vi "Main.vi"(11 "Module Admin":refnum<class "Delacor_lib_QMH_Module Admin.lvclass">) -> ()   [LabVIEW 2020, in "Topas.lvlib"]
doc: "This template is based off of the Queued Message Handler design pattern and the Queued Message Handler project template that ships with LabVIEW.\n\nThe main difference is that the queue is private to this module and communication between modules is performed via Broadcast and Request events.\n\nRequest events are wrapped in public API methods and are handled in the Event Handling Loop (EHL) of this VI. Any module can register for Broadcast events sent by this module. The EHL generates messages based on user interface actions.\n\nThe Message Handling Loop (MHL) processes messages generated by the EHL, or by other messages. The messages are string values, so new messages can be added easily to the Message Cases case structure in the MHL. Each message cluster can also provide an optional value for Message Data, which is a variant that can be converted to whatever message-specific data is required.\n_____\nBased on Delacor QMH Project Template 5.0.0.82."
uses:
  Topas.lvlib
  <vilib>/Delacor/Delacor QMH/Libraries/Module Admin_class/Delacor_lib_QMH_Module Admin.lvclass
  Module Data--cluster.ctl
  Topas-LVClass/Abstract Topas/Abstract Topas.lvclass
  Stop Argument--cluster.ctl
  <vilib>/Delacor/Delacor QMH/Libraries/Message Queue_class/Delacor_lib_QMH_Message Queue.lvclass/Delacor_lib_QMH_Message Queue.ctl
  <vilib>/Delacor/Delacor QMH/Libraries/Module Admin_class/Delacor_lib_QMH_Module Admin.lvclass/Delacor_lib_QMH_Module Admin.ctl
  Set Wavelength Argument--cluster.ctl
  Set Wavelength (Reply Payload)--cluster.ctl
  Open Shutter Argument--cluster.ctl
  Get Wavelength Argument--cluster.ctl
  Get Wavelength (Reply Payload)--cluster.ctl
  Get Module Data Argument--cluster.ctl
  Get Module Data (Reply Payload)--cluster.ctl
  <vilib>/Utility/miscctls.llb/LVPointTypeDef.ctl
  <vilib>/Delacor/Delacor QMH/Libraries/Message Queue_class/Delacor_lib_QMH_Enqueue Message (Single).vi
  <vilib>/Delacor/Delacor QMH/Libraries/Module Admin_class/Delacor_lib_QMH_Get External Launch.vi
  <vilib>/Utility/error.llb/Error Cluster From Error Code.vi
  <vilib>/ErrorRing/Error Ring.xnode
  <vilib>/Delacor/Delacor QMH/Libraries/Message Queue_class/Delacor_lib_QMH_Message Queue.lvclass
panel:
  out "error out":errorcluster
  out "Status":string
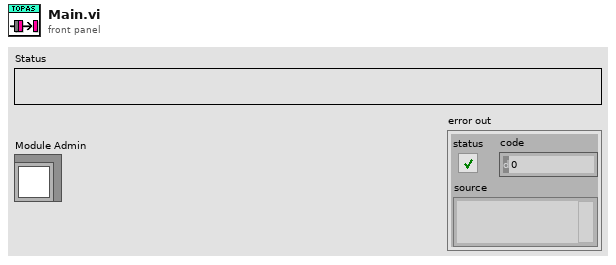
[diagram p1: front panel]
types:
  T1 = typedef "Topas.lvlib/Request Events--cluster.ctl" = cluster{"Stop Module":refnum<user-event>, "Show Panel":refnum<user-event>, "Hide Panel":refnum<user-event>, "Get Module Execution Status":refnum<user-event>, "Show Diagram":refnum<user-event>, "Set Wavelength":refnum<user-event>, "Open Shutter":refnum<user-event>, "Get Wavelength":refnum<user-event>, "Get Module Data":refnum<user-event>}
  T2 = typedef "Topas.lvlib/Module Data--cluster.ctl" = cluster{"Status":string, "Wavelength":dbl, "-Topas Class":refnum<class "Abstract Topas.lvclass">}
  T3 = enum32{"invalid lock state", "Not Locked", "Locked (No Password)", "Password-protected"}
  T4 = typedef "Topas.lvlib/Stop Argument--cluster.ctl" = cluster{"Origin":string, "Exit via Stop Module Req?":bool, "Wait for Module to stop?":bool}
  T5 = typedef "Topas.lvlib/Set Wavelength Argument--cluster.ctl" = cluster{"Wavelength":dbl, "Wait Notifier":refnum<notifier>, "wait for reply":bool}
  T6 = typedef "Topas.lvlib/Open Shutter Argument--cluster.ctl" = cluster{"Open Shutter":bool}
  T7 = typedef "Topas.lvlib/Get Wavelength Argument--cluster.ctl" = cluster{"Wait Notifier":refnum<notifier>, "wait for reply":bool}
  T8 = typedef "Topas.lvlib/Get Module Data Argument--cluster.ctl" = cluster{"Wait Notifier":refnum<notifier>, "wait for reply":bool}
  T9 = typedef "LVPointTypeDef.ctl" = cluster{"Horizontal":i16, "Vertical":i16}
  T10 = enum32{"Invalid", "Standard", "Closed", "Hidden", "Minimized", "Maximized"}
  T11 = typedef "Topas.lvlib/Set Wavelength (Reply Payload)--cluster.ctl" = cluster{"Wavelength":dbl, "Set Wavelength_error":errorcluster}
  T12 = typedef "Topas.lvlib/Get Wavelength (Reply Payload)--cluster.ctl" = cluster{"Wavelength":dbl, "Get Wavelength_error":errorcluster}
  T13 = typedef "Topas.lvlib/Get Module Data (Reply Payload)--cluster.ctl" = cluster{"Topas":T2, "Get Module Data_error":errorcluster}
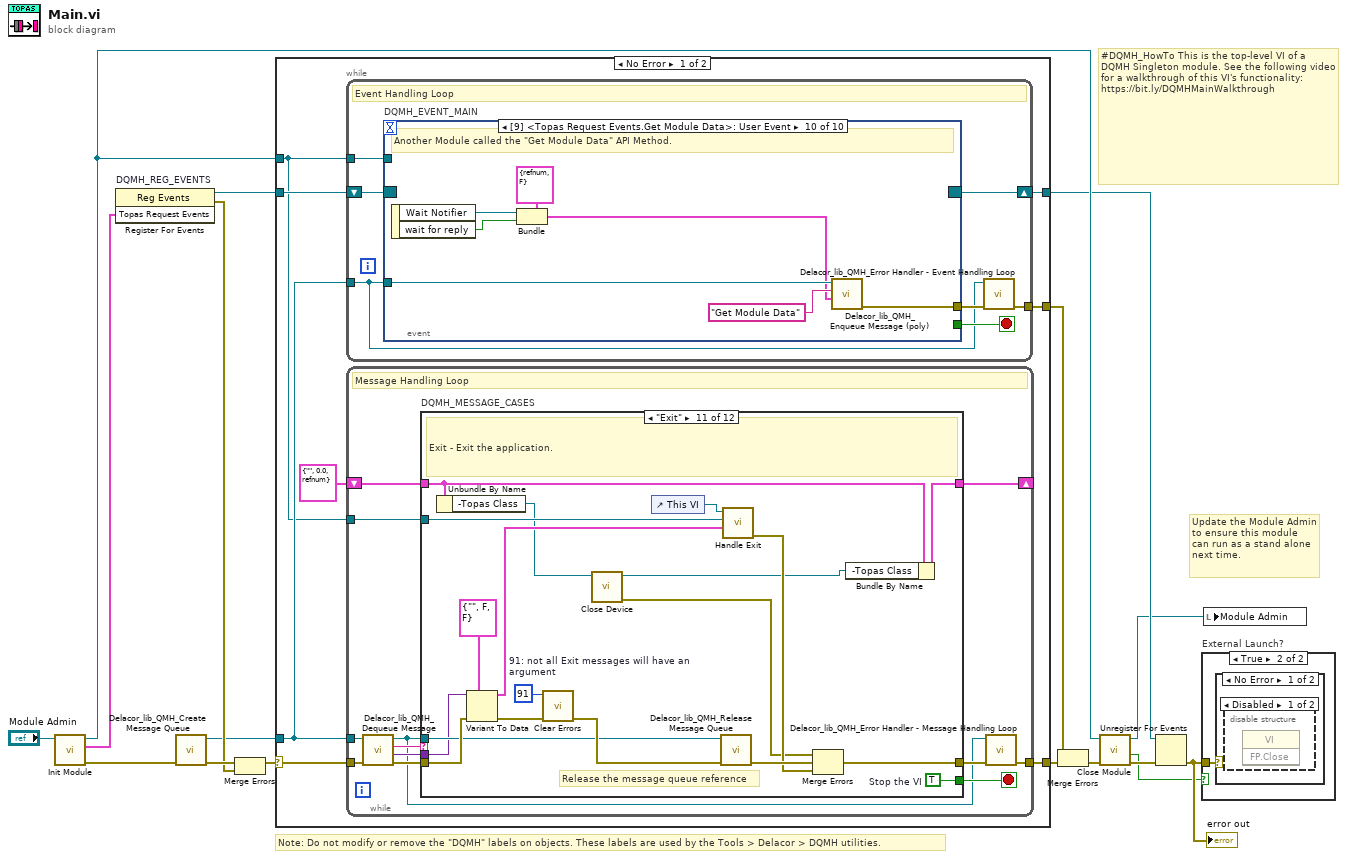
[diagram p0: block diagram]
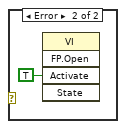
[diagram p4: hidden frame]
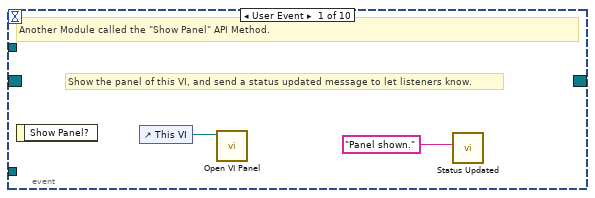
[diagram p5: hidden frame]
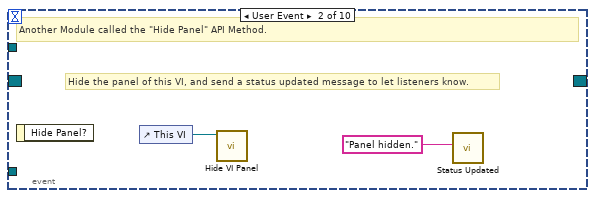
[diagram p6: hidden frame]
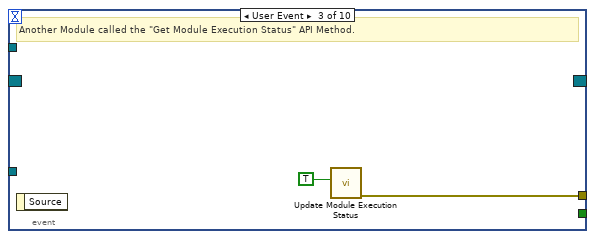
[diagram p7: hidden frame]
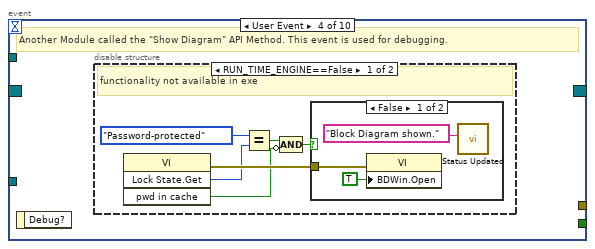
[diagram p8: hidden frame]
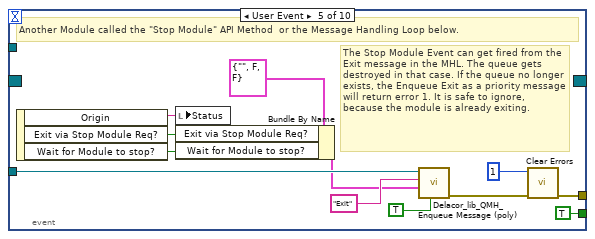
[diagram p11: hidden frame]
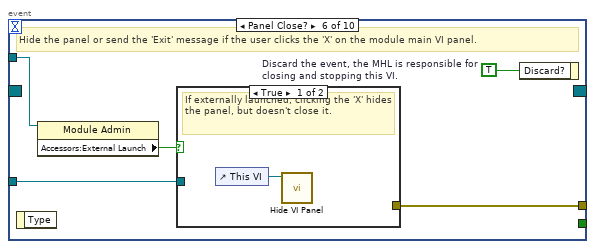
[diagram p12: hidden frame]
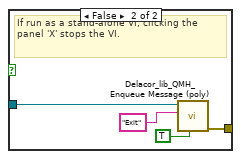
[diagram p13: hidden frame]
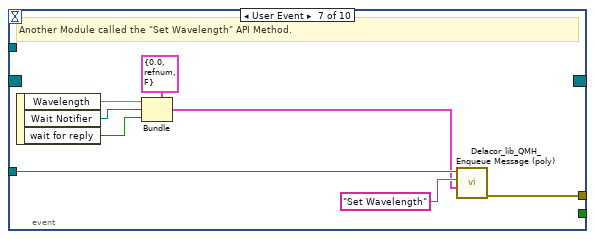
[diagram p14: hidden frame]
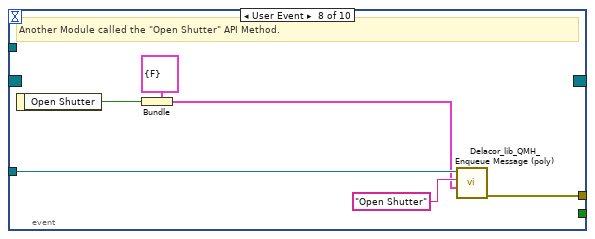
[diagram p15: hidden frame]
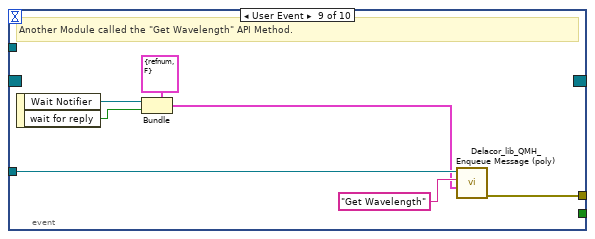
[diagram p16: hidden frame]
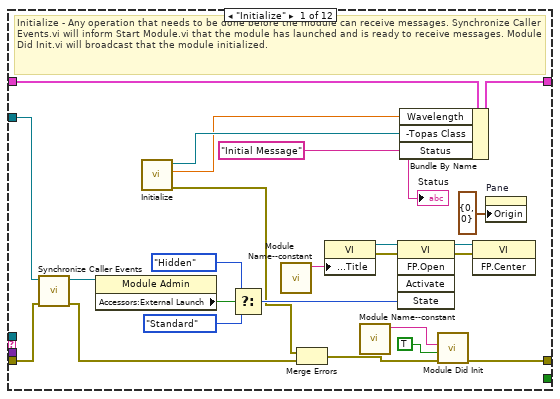
[diagram p17: hidden frame]
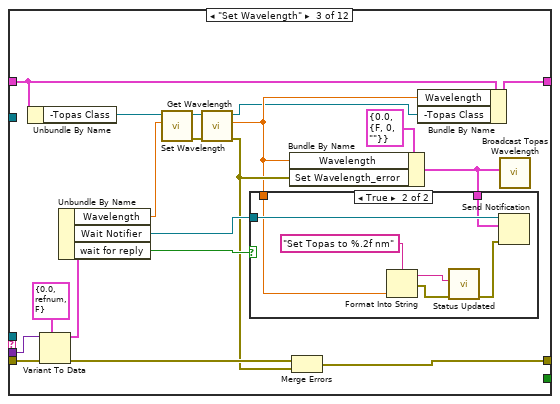
[diagram p19: hidden frame]
diagram:
  # "#DQMH_HowTo This is the top-level VI of a DQMH Singleton module. See the following video for a walkthrough of this VI's functionality: https://bit.ly/DQMHMainWalkthrough"
  # "Note: Do not modify or remove the \"DQMH\" labels on objects. These labels are used by the Tools > Delacor > DQMH utilities."
  # "Update the Module Admin to ensure this module can run as a stand alone next time."
  n1 = call "Init Module.vi"("Singleton Module Admin in"="Module Admin") -> ("error out"=w16:errorcluster, "Topas Request Events"=w5:T1, "Singleton Module Admin out"=w8:refnum<class "Delacor_lib_QMH_Module Admin.lvclass">)  [unwired: 8 in]
  n2 = register-events "DQMH_REG_EVENTS"(w5) -> (reference out=w6:refnum<event-registration>, error out=w9:errorcluster)  [unwired: 2 in]
  n3 = call <vilib>:"Delacor_lib_QMH_Create Message Queue.vi"("error in (no error)"=w16) -> ("error out"=w11:errorcluster, "Message Queue"=w4:refnum<class "Delacor_lib_QMH_Message Queue.lvclass">)  [unwired: 9 in]
  n4 = Merge Errors(w11, w9) -> (w10:errorcluster)
  n5 = case shown="No Error" w10 {
    selector: w10 -> [w23 w275]
    tunnel: [w25 w274] -> w17
    tunnel: [w22 w280] -> w7
    tunnel: w6 -> [w20 w280]
    tunnel: w4 -> [w19 w273]
    tunnel: [w24 _] -> w14
    tunnel: w8 -> [w18 w276]
    frame No Error {
      n6 = while {
        tunnel: w19 -> [w26]
        shift-right: [w29] -> w22
        shift-left: w20 -> [w30]
        tunnel: [w31] -> w24
        tunnel: w18 -> [w27]
        stop <- w28 stop-if-true
        # "Event Handling Loop"
        n7 = event "DQMH_EVENT_MAIN" shown="[9] <Topas Request Events.Get Module Data>: User Event" {
          selector: w30 -> [_ _ _ _ _ _ _ _ _ _]
          dyn-events: [_ _ _ _ _ _ _ _ _ _] -> w29
          timeout: _ -> [_ _ _ _ _ _ _ _ _ _]
          tunnel: [_ _ _ _ TRUE ("Discard?") _ _ _ _ _] -> w28
          tunnel: w26 -> [_ _ _ _ w55 w62 w77 w83 w90 w97]
          tunnel: [_ _ w38 _ w58 w64 w70 w78 w84 w91] -> w32
          tunnel: w27 -> [_ _ _ _ _ w61 _ _ _ _]
          event User Event {
            # "Show the panel of this VI, and send a status updated message to let listeners know."
            # "Another Module called the \"Show Panel\" API Method."
            n8 = event-data() -> ()  [unwired: 1 in, 1 out]
            n9 = control-ref of="This VI"() -> (w34:refnum<vi>)
            n10 = call "Open VI Panel.vi"("VI"=w34) -> ()  [unwired: 10 in, 1 out]
            n11 = call "Status Updated.vi"("Status"="Panel shown." ("format string")) -> ()  [unwired: 10 in, 1 out]
          }
          event User Event {
            # "Hide the panel of this VI, and send a status updated message to let listeners know."
            # "Another Module called the \"Hide Panel\" API Method."
            n12 = event-data() -> ()  [unwired: 1 in, 1 out]
            n13 = control-ref of="This VI"() -> (w36:refnum<vi>)
            n14 = call "Hide VI Panel.vi"("VI"=w36) -> ()  [unwired: 10 in, 1 out]
            n15 = call "Status Updated.vi"("Status"="Panel hidden." ("format string")) -> ()  [unwired: 10 in, 1 out]
          }
          event User Event {
            # "Another Module called the \"Get Module Execution Status\" API Method."
            n16 = event-data() -> ()  [unwired: 1 in, 1 out]
            n17 = call "Update Module Execution Status.vi"("Running?"=TRUE) -> ("error out"=w38:errorcluster)  [unwired: 10 in]
          }
          event User Event {
            # "Another Module called the \"Show Diagram\" API Method. This event is used for debugging."
            n18 = event-data() -> ()  [unwired: 1 in, 1 out]
            n19 = disable-structure shown="RUN_TIME_ENGINE==False" {
              frame condition #0 (active) {
                # "functionality not available in exe"
                n20 = invoke class="VI" method="Lock State.Get"() -> (error out=w44:errorcluster, "Get Lock State"=w43:T3, "pwd in cache"=w40:bool)  [unwired: 4 in, 1 out]
                n21 = Equal?(x=T3."Password-protected", y=w43) -> (x = y?=w41:bool)
                n22 = Compound Arithmetic op=AND(w41, invert w40) -> (w39:bool)
                n23 = case shown="False" w39 {
                  tunnel: w44 -> [w47 _]
                  frame False {
                    n24 = property class="VI"(error in=w47, "BDWin.Open"=TRUE ("Block Diagram Window:Open")) -> ()  [unwired: 1 in, 2 out]
                    n25 = call "Status Updated.vi"("Status"="Block Diagram shown." ("format string")) -> ()  [unwired: 10 in, 1 out]
                  }
                  frame True {
                    # "Password-protected VI, and the password is not in the cache. Do not show the diagram."
                  }
                }
              }
              frame condition #1 {
              }
            }
          }
          event User Event {
            # "The Stop Module Event can get fired from the Exit message in the MHL. The queue gets destroyed in that case. If the queue no longer exists, the Enqueue Exit as a priority message will return error 1. It is safe to ignore, because the module is already exiting."
            # "Another Module called the \"Stop Module\" API Method  or the Message Handling Loop below."
            n26 = event-data() -> ("Origin"=w54:string, "Exit via Stop Module Req?"=w50:bool, "Wait for Module to stop?"=w49:bool)  [unwired: 1 in]
            n27 = local write "Status"(w54) -> ()
            n28 = Bundle By Name(cluster=T4 {"Origin"="", "Exit via Stop Module Req?"=FALSE, "Wait for Module to stop?"=FALSE} ("Stop Argument"), "Exit via Stop Module Req?"=w50, "Wait for Module to stop?"=w49) -> (w48:T4)
            n29 = call-poly <vilib>:"Delacor_lib_QMH_Enqueue Message (poly).vi"("Priority Message? (F)"=TRUE, "Message Data"=w48, "Message"="Exit", "Message Queue in"=w55) -> ("error out"=w59:errorcluster)  [unwired: 6 in, 1 out]
            n30 = call <vilib>:"Clear Errors.vi"("error in (no error)"=w59, "specific error code to clear (0: all)"=1) -> ("error out"=w58:errorcluster)  [unwired: 4 in, 1 out]
          }
          event Panel Close? {
            w63 = TRUE  # Discard the event, the MHL is responsible for closing and stopping this VI.
            # "Hide the panel or send the 'Exit' message if the user clicks the 'X' on the module main VI panel."
            n31 = event-data() -> ()  [unwired: 1 in, 1 out]
            n32 = property class="Module Admin"(reference=w61) -> ("Accessors:External Launch"=w60:bool)  [unwired: 1 in, 2 out]
            n33 = case shown="True" w60 {
              tunnel: w62 -> [_ w68]
              tunnel: [_ w69] -> w64
              frame True {
                # "If externally launched, clicking the 'X' hides the panel, but doesn't close it."
                n34 = control-ref of="This VI"() -> (w65:refnum<vi>)
                n35 = call "Hide VI Panel.vi"("VI"=w65) -> ()  [unwired: 10 in, 1 out]
              }
              frame False {
                # "If run as a stand-alone VI, clicking the panel 'X' stops the VI."
                n36 = call-poly <vilib>:"Delacor_lib_QMH_Enqueue Message (poly).vi"("Priority Message? (F)"=TRUE, "Message"="Exit", "Message Queue in"=w68) -> ("error out"=w69:errorcluster)  [unwired: 7 in, 1 out]
              }
            }
            n37 = event-data("Discard?"=w63) -> ()  [unwired: 1 in, 1 out]
          }
          event User Event {
            # "Another Module called the \"Set Wavelength\" API Method."
            n38 = event-data() -> ("Wavelength"=w73:dbl, "Wait Notifier"=w72:refnum<notifier>, "wait for reply"=w71:bool)  [unwired: 1 in]
            n39 = Bundle(cluster=T5 {"Wavelength"=0.0, "Wait Notifier"=refnum, "wait for reply"=FALSE} ("Set Wavelength Argument"), "Wavelength"=w73, "Wait Notifier"=w72, "wait for reply"=w71) -> (w74:T5)
            n40 = call-poly <vilib>:"Delacor_lib_QMH_Enqueue Message (poly).vi"("Message Data"=w74, "Message"="Set Wavelength", "Message Queue in"=w77) -> ("error out"=w70:errorcluster)  [unwired: 7 in, 1 out]
          }
          event User Event {
            # "Another Module called the \"Open Shutter\" API Method."
            n41 = event-data() -> ("Open Shutter"=w79:bool)  [unwired: 1 in]
            n42 = Bundle(cluster=T6 {"Open Shutter"=FALSE} ("Open Shutter Argument"), "Open Shutter"=w79) -> (w80:T6)
            n43 = call-poly <vilib>:"Delacor_lib_QMH_Enqueue Message (poly).vi"("Message Data"=w80, "Message"="Open Shutter", "Message Queue in"=w83) -> ("error out"=w78:errorcluster)  [unwired: 7 in, 1 out]
          }
          event User Event {
            # "Another Module called the \"Get Wavelength\" API Method."
            n44 = event-data() -> ("Wait Notifier"=w86:refnum<notifier>, "wait for reply"=w85:bool)  [unwired: 1 in]
            n45 = Bundle(cluster=T7 {"Wait Notifier"=refnum, "wait for reply"=FALSE} ("Get Wavelength Argument"), "Wait Notifier"=w86, "wait for reply"=w85) -> (w87:T7)
            n46 = call-poly <vilib>:"Delacor_lib_QMH_Enqueue Message (poly).vi"("Message Data"=w87, "Message"="Get Wavelength", "Message Queue in"=w90) -> ("error out"=w84:errorcluster)  [unwired: 7 in, 1 out]
          }
          event User Event {
            # "Another Module called the \"Get Module Data\" API Method."
            n47 = event-data() -> ("Wait Notifier"=w93:refnum<notifier>, "wait for reply"=w92:bool)  [unwired: 1 in]
            n48 = Bundle(cluster=T8 {"Wait Notifier"=refnum, "wait for reply"=FALSE} ("Get Module Data Argument"), "Wait Notifier"=w93, "wait for reply"=w92) -> (w94:T8)
            n49 = call-poly <vilib>:"Delacor_lib_QMH_Enqueue Message (poly).vi"("Message Data"=w94, "Message"="Get Module Data", "Message Queue in"=w97) -> ("error out"=w91:errorcluster)  [unwired: 7 in, 1 out]
          }
        }
        n50 = call-dynamic "Delacor_lib_QMH_Error Handler - Event Handling Loop.vi"("error in (no error)"=w32, "Message Queue in"=w26) -> ("dup error in"=w31:errorcluster)  [unwired: 8 in, 1 out]
      }
      n51 = while {
        tunnel: w19 -> [w100]
        shift-right: [w104] -> _
        shift-left: T2 {"Status"="", "Wavelength"=0.0, "-Topas Class"=refnum} ("Data Cluster") -> [w105]
        tunnel: w23 -> [w108]
        tunnel: [w106] -> w25
        tunnel: w18 -> [w98]
        stop <- w103 stop-if-true
        # "Message Handling Loop"
        n52 = call-dynamic "Delacor_lib_QMH_Dequeue Message.vi"("error in (no error)"=w108, "Message Queue in"=w100) -> ("error out"=w107:errorcluster, "Message Data"=w101:variant, "Message"=w102:string, "Message Queue out"=w99:refnum<class "Delacor_lib_QMH_Message Queue.lvclass">)  [unwired: 6 in]
        n53 = case "DQMH_MESSAGE_CASES" shown="\"Exit\"" w102 {
          selector: w102 -> [_ _ _ _ _ _ _ _ _ _ _ w260]
          tunnel: w99 -> [_ _ _ _ _ _ _ _ _ w226 w252 _]
          tunnel: w107 -> [w131 w135 w154 w173 w189 w203 w208 w210 w215 w233 w258 w262]
          tunnel: [w129 w135 w145 w165 w180 w194 w207 w210 w214 w229 w255 w263] -> w109
          tunnel: w105 -> [w120 w134 w144 w167 w179 w193 w206 w209 w212 w228 w243 w261]
          tunnel: [w119 w134 w138 w163 w176 w193 w206 w209 w212 w228 w241 w261] -> w104
          tunnel: [_ _ _ _ _ _ _ _ _ _ w251 _] -> w103
          tunnel: w101 -> [_ _ w152 w171 w187 w201 _ _ _ w227 w250 _]
          tunnel: w98 -> [w121 _ _ _ _ _ _ _ _ w225 w245 _]
          frame "Initialize" {
            w114 = "Initial Message" ("Initial Message")
            # "Initialize - Any operation that needs to be done before the module can receive messages. Synchronize Caller Events.vi will inform Start Module.vi that the module has launched and is ready to receive messages. Module Did Init.vi will broadcast that the module initialized."
            n54 = call "Synchronize Caller Events.vi"("error in (no error)"=w131, "Singleton Module Admin in"=w121) -> ("error out"=w130:errorcluster, "Singleton Module Admin out"=w116:refnum<class "Delacor_lib_QMH_Module Admin.lvclass">)  [unwired: 8 in]
            n55 = property class="Module Admin"(reference=w116) -> ("Accessors:External Launch"=w125:bool)  [unwired: 1 in, 2 out]
            n56 = call "Initialize.vi"() -> ("error out"=w112:errorcluster, "Wavelength"=w110:dbl, "Abstract Topas out"=w111:refnum<class "Abstract Topas.lvclass">)  [unwired: 9 in]
            n57 = Select(t=T10."Hidden" ("State"), s=w125, f=T10."Standard" ("State")) -> (s? t:f=w122:T10)
            n58 = call "Module Name--constant.vi"() -> ("Module Name"=w128:string)  [unwired: 11 in]
            n59 = Merge Errors(w112, w130) -> (w113:errorcluster)
            n60 = property class="VI"("Front Panel.Title"=w128) -> (reference out=w127:refnum<vi>, error out=w133:errorcluster)  [unwired: 2 in]
            n61 = call "Module Name--constant.vi"() -> ("Module Name"=w117:string)  [unwired: 11 in]
            n62 = invoke class="VI" method="FP.Open"(reference=w127, error in=w133, "State"=w122) -> (reference out=w126:refnum<vi>, error out=w132:errorcluster)  [unwired: 2 in, 3 out]
            n63 = Bundle By Name(cluster=w120, "Wavelength"=w110, "-Topas Class"=w111, "Status"=w114) -> (w119:T2)
            n64 = call "Module Did Init.vi"("error in (no error)"=w113, "Initialized?"=TRUE, "Origin"=w117) -> ("error out"=w129:errorcluster)  [unwired: 8 in]
            n65 = invoke class="VI" method="FP.Center"(reference=w126, error in=w132) -> ()  [unwired: 1 in, 3 out]
            n66 = property on="Pane" class="Pane"("Origin"=T9 {"Horizontal"=0, "Vertical"=0}) -> ()  [unwired: 2 in, 2 out]
            "Status" <- w114
          }
          frame "--- Module Specific ---" {
            # "Separator -- The following cases handle messages specific to this Module."
          }
          frame "Set Wavelength" {
            n67 = Unbundle By Name(w144) -> ("-Topas Class"=w143:refnum<class "Abstract Topas.lvclass">)
            n68 = Variant To Data(error in=w154, type=T5 {"Wavelength"=0.0, "Wait Notifier"=refnum, "wait for reply"=FALSE} ("Set Wavelength Argument"), Variant=w152) -> (data=w150:T5, error out=w153:errorcluster)
            n69 = Unbundle By Name(w150) -> ("Wavelength"=w140:dbl, "Wait Notifier"=w149:refnum<notifier>, "wait for reply"=w148:bool)
            n70 = call-dynamic "Set Wavelength.vi"("Wavelength"=w140, "Abstract Topas in"=w143) -> ("error out"=w142:errorcluster, "Abstract Topas out"=w141:refnum<class "Abstract Topas.lvclass">)  [unwired: 8 in]
            n71 = call-dynamic "Get Wavelength.vi"("error in (no error)"=w142, "Abstract Topas in"=w141) -> ("error out"=w139:errorcluster, "Wavelength"=w137:dbl, "Abstract Topas out"=w136:refnum<class "Abstract Topas.lvclass">)  [unwired: 7 in]
            n72 = Bundle By Name(cluster=T11 {"Wavelength"=0.0, "Set Wavelength_error"={"status"=FALSE, "code"=0, "source"=""}} ("Set Wavelength (Reply Payload)"), "Wavelength"=w137, "Set Wavelength_error"=w139) -> (w147:T11)
            n73 = case shown="True" w148 {
              tunnel: w149 -> [_ w161]
              tunnel: w147 -> [_ w160]
              tunnel: w137 -> [_ w156]
              frame False {
              }
              frame True {
                n74 = Format Into String(format string="Set Topas to %.2f nm", w156) -> (resulting string=w157:string, error out=w158:errorcluster)  [unwired: 2 in]
                n75 = call "Status Updated.vi"("error in (no error)"=w158, "Status"=w157) -> ("error out"=w159:errorcluster)  [unwired: 9 in]
                n76 = Send Notification(notification=w160, notifier=w161, error in (no error)=w159) -> ()  [unwired: 2 out]
              }
            }
            n77 = Merge Errors(w153, w139) -> (w145:errorcluster)
            n78 = Bundle By Name(cluster=w144, "Wavelength"=w137, "-Topas Class"=w136) -> (w138:T2)
            n79 = call "Broadcast Topas Wavelength.vi"("Reply Payload"=w147) -> ()  [unwired: 10 in, 1 out]
          }
          frame "Open Shutter" {
            # "Passing True opens the shutter, False closes it."
            n80 = Variant To Data(error in=w173, type=T6 {"Open Shutter"=FALSE} ("Open Shutter Argument"), Variant=w171) -> (data=w169:T6, error out=w172:errorcluster)
            n81 = Unbundle By Name(w167) -> ("-Topas Class"=w166:refnum<class "Abstract Topas.lvclass">)
            n82 = Unbundle By Name(w169) -> ("Open Shutter"=w168:bool)
            n83 = call-dynamic "Open Shutter.vi"("Open Shutter"=w168, "Abstract Topas in"=w166) -> ("error out"=w164:errorcluster, "Abstract Topas out"=w162:refnum<class "Abstract Topas.lvclass">)  [unwired: 8 in]
            n84 = Merge Errors(w164, w172) -> (w165:errorcluster)
            n85 = Bundle By Name(cluster=w167, "-Topas Class"=w162) -> (w163:T2)
          }
          frame "Get Wavelength" {
            # "Get the wavelength in nm"
            n86 = Variant To Data(error in=w189, type=T7 {"Wait Notifier"=refnum, "wait for reply"=FALSE} ("Get Wavelength Argument"), Variant=w187) -> (data=w185:T7, error out=w188:errorcluster)
            n87 = Unbundle By Name(w179) -> ("-Topas Class"=w178:refnum<class "Abstract Topas.lvclass">)
            n88 = Unbundle By Name(w185) -> ("Wait Notifier"=w184:refnum<notifier>, "wait for reply"=w183:bool)
            n89 = call-dynamic "Get Wavelength.vi"("Abstract Topas in"=w178) -> ("error out"=w177:errorcluster, "Wavelength"=w175:dbl, "Abstract Topas out"=w174:refnum<class "Abstract Topas.lvclass">)  [unwired: 8 in]
            n90 = Bundle By Name(cluster=w179, "Wavelength"=w175, "-Topas Class"=w174) -> (w176:T2)
            n91 = Bundle By Name(cluster=T12 {"Wavelength"=0.0, "Get Wavelength_error"={"status"=FALSE, "code"=0, "source"=""}} ("Get Wavelength (Reply Payload)"), "Wavelength"=w175, "Get Wavelength_error"=w177) -> (w182:T12)
            n92 = case shown="True" w183 {
              tunnel: w184 -> [_ w191]
              tunnel: w182 -> [_ w190]
              frame False {
              }
              frame True {
                n93 = Send Notification(notification=w190, notifier=w191) -> ()  [unwired: 1 in, 2 out]
              }
            }
            n94 = Merge Errors(w188) -> (w180:errorcluster)
          }
          frame "Get Module Data" {
            n95 = Variant To Data(error in=w203, type=T8 {"Wait Notifier"=refnum, "wait for reply"=FALSE} ("Get Module Data Argument"), Variant=w201) -> (data=w199:T8, error out=w202:errorcluster)
            n96 = Unbundle By Name(w199) -> ("Wait Notifier"=w198:refnum<notifier>, "wait for reply"=w197:bool)
            n97 = Bundle By Name(cluster=T13 {"Topas"={"Status"="", "Wavelength"=0.0, "-Topas Class"=refnum}, "Get Module Data_error"={"status"=FALSE, "code"=0, "source"=""}} ("Get Module Data (Reply Payload)"), "Topas"=w193, "Get Module Data_error"=errorcluster {"status"=FALSE, "code"=0, "source"=""}) -> (w196:T13)
            n98 = case shown="True" w197 {
              tunnel: w198 -> [_ w205]
              tunnel: w196 -> [_ w204]
              frame False {
              }
              frame True {
                n99 = Send Notification(notification=w204, notifier=w205) -> ()  [unwired: 1 in, 2 out]
              }
            }
            n100 = Merge Errors(w202) -> (w194:errorcluster)
          }
          frame "---Copy This Frame---" {
            # "Duplicate this frame when creating new messages.  Change this comment in the duplicated frame to describe this message."
            n101 = Merge Errors(w208) -> (w207:errorcluster)
          }
          frame "--- Exit and Error Handling---" {
            # "Separator - The following cases handle errors and exit messages."
          }
          frame "Simulate MHL Error" {
            # "#DQMH_HowTo The 'Simulate MHL Error' button  illustrates how the MHL handles errors. This event is instructional in nature and can be removed."
            # "Simulate an error occurring at the MHL"
            n102 = call "Module Name--constant.vi"() -> ("Module Name"=w211:string)  [unwired: 11 in]
            n103 = xnode "Error Ring"("parameter 0"=w211) -> ("error out"=w213:errorcluster)
            n104 = Merge Errors(w215, w213) -> (w214:errorcluster)
          }
          frame "Error" {
            # "#CodeRecommended - If you ever change the name of this \"Error\" message, you'll need to update the name in the Check Loop Error.vi as well."
            # "#CodeRecommended - If the module is running in standalone mode (External Launch = FALSE), this code will pop up an error dialog and call the 'Exit' message if an error occurs. Add more fine-grained error handling here."
            # "Error - Check the error message data and respond accordingly. This message is sent by the \"Error Handler\" VIs at the end of each loop in this application."
            n105 = property class="Module Admin"(reference=w225) -> ("Accessors:External Launch"=w224:bool)  [unwired: 1 in, 2 out]
            n106 = Variant To Data(error in=w233, type=errorcluster {"status"=FALSE, "code"=0, "source"=""} ("error constant"), Variant=w227) -> (data=w234:errorcluster, error out=w231:errorcluster)
            n107 = call "Module Name--constant.vi"() -> ("Module Name"=w223:string)  [unwired: 11 in]
            n108 = call "Error Reported.vi"("Additional Information"=w223, "Error"=w234) -> ()  [unwired: 9 in, 1 out]
            n109 = case shown="False" w224 {
              tunnel: [w239 _] -> w230
              tunnel: w226 -> [w237 _]
              tunnel: w234 -> [w238 _]
              frame False {
                # "If the module is running standalone, then pop up an error dialog and call the \"Exit\" message."
                n110 = call <vilib>:"Simple Error Handler.vi"("error in (no error)"=w238) -> ()  [unwired: 4 in, 5 out]
                n111 = call-poly <vilib>:"Delacor_lib_QMH_Enqueue Message (poly).vi"("Priority Message? (F)"=TRUE, "Message"="Exit", "Message Queue in"=w237) -> ("error out"=w239:errorcluster)  [unwired: 7 in, 1 out]
              }
              frame True {
                # "If the module was launched externally, calling the Error Reported broadcast VI is the only action performed by the \"Error\" message. The module's caller can then process the error appropriately."
              }
            }
            n112 = Merge Errors(w231, w230) -> (w229:errorcluster)
            n113 = local write "error out"(w229) -> ()
          }
          frame "Exit" {
            w249 = 91  # 91: not all Exit messages will have an argument
            w251 = TRUE  # Stop the VI
            # "Release the message queue reference"
            # "Exit - Exit the application."
            n114 = Unbundle By Name(w243) -> ("-Topas Class"=w242:refnum<class "Abstract Topas.lvclass">)
            n115 = Variant To Data(error in=w258, type=T4 {"Origin"="", "Exit via Stop Module Req?"=FALSE, "Wait for Module to stop?"=FALSE} ("Stop Argument"), Variant=w250) -> (data=w247:T4, error out=w254:errorcluster)
            n116 = call <vilib>:"Clear Errors.vi"("error in (no error)"=w254, "specific error code to clear (0: all)"=w249) -> ("error out"=w257:errorcluster)  [unwired: 4 in, 1 out]
            n117 = call-dynamic "Close Device.vi"("Abstract Topas in"=w242) -> ("error out"=w244:errorcluster, "Abstract Topas out"=w240:refnum<class "Abstract Topas.lvclass">)  [unwired: 9 in]
            n118 = control-ref of="This VI"() -> (w246:refnum<vi>)
            n119 = call-dynamic "Delacor_lib_QMH_Release Message Queue.vi"("error in (no error)"=w257, "Message Queue"=w252) -> ("error out"=w256:errorcluster)  [unwired: 9 in]
            n120 = call "Handle Exit.vi"("Stop Argument"=w247, "Admin in"=w245, "VI reference"=w246) -> ("error out"=w253:errorcluster)  [unwired: 7 in, 1 out]
            n121 = Merge Errors(w244, w256, w253) -> (w255:errorcluster)
            n122 = Bundle By Name(cluster=w243, "-Topas Class"=w240) -> (w241:T2)
          }
          frame Default {
            # "'Default' case only runs if there is a message that isn't defined in any of the other cases.  Output a programming error."
            n123 = call "Module Name--constant.vi"() -> ("Module Name"=w259:string)  [unwired: 11 in]
            n124 = xnode "Error Ring"("parameter 0"=w260, "parameter 1"=w259) -> ("error out"=w264:errorcluster)
            n125 = Merge Errors(w262, w264) -> (w263:errorcluster)
          }
        }
        n126 = call-dynamic "Delacor_lib_QMH_Error Handler - Message Handling Loop.vi"("error in (no error)"=w109, "Message Queue in"=w99) -> ("dup error in"=w106:errorcluster)  [unwired: 8 in, 1 out]
      }
    }
    frame Error {
      # "Synchronize Caller Events.vi will inform Start Module.vi that the module has launched and will let the code calling Start Module.vi register for broadcasts and would permit the caller receive the broadcast that an error occurred at launch time."
      n127 = call-dynamic "Delacor_lib_QMH_Release Message Queue.vi"("error in (no error)"=w275, "Message Queue"=w273) -> ("error out"=w274:errorcluster)  [unwired: 9 in]
      n128 = call "Synchronize Caller Events.vi"("Singleton Module Admin in"=w276) -> ("error out"=w281:errorcluster)  [unwired: 9 in, 1 out]
      n129 = call "Module Name--constant.vi"() -> ("Module Name"=w279:string)  [unwired: 11 in]
      n130 = Format Into String(format string="An error occurred during initialization. %s is no longer running.", w279) -> (resulting string=w277:string)  [unwired: 2 in, 1 out]
      n131 = Merge Errors(w274, w281) -> (w282:errorcluster)
      n132 = call "Error Reported.vi"("Additional Information"=w277, "Error"=w282) -> ()  [unwired: 9 in, 1 out]
    }
  }
  n133 = Merge Errors(w14, w17) -> (w13:errorcluster)
  n134 = call "Close Module.vi"("error in (no error)"=w13, "Module Admin in"=w8) -> ("error out"=w15:errorcluster, "External Launch"=w1:bool, "Module Admin out"=w2:refnum<class "Delacor_lib_QMH_Module Admin.lvclass">)  [unwired: 7 in]
  n135 = Unregister For Events(event registration refnum=w7, error in=w15) -> (error out=w12:errorcluster)
  "error out" <- w12
  n136 = case "External Launch?" shown="True" w1 {
    tunnel: w12 -> [_ w283]
    frame False {
    }
    frame True {
      n137 = case shown="No Error" w283 {
        frame No Error {
          n138 = disable-structure shown="Disabled" {
            frame Disabled {
              n139 = invoke class="VI" method="FP.Close"() -> ()  [unwired: 3 in, 3 out]
            }
            frame Enabled {
            }
          }
        }
        frame Error {
          n140 = invoke class="VI" method="FP.Open"("Activate"=TRUE ("Activate?")) -> ()  [unwired: 4 in, 5 out]
        }
      }
    }
  }
  n141 = local write "Module Admin"(w2) -> ()
